vi "Initialize.vi"(0 "ToneCloud in":refnum<class "Tone Cloud.lvclass">, 1 "Filter in":refnum<class "Filter.lvclass">, 5 "Level in":refnum<class "Level.lvclass">, 7 "Fs (Hz)":dbl, 9 "Npts":i32, 11 "error in (no error)":errorcluster, 13 "Channel Name":string) -> (3 "Filter out":refnum<class "Filter.lvclass">, 4 "ToneCloud out":refnum<class "Tone Cloud.lvclass">, 6 "Level out":refnum<class "Level.lvclass">, 15 "error out":errorcluster)   [LabVIEW 2020, in "Tone Cloud.lvclass"]
uses:
  Tone Cloud.lvclass
  Level/Level.lvclass
  Filter/Filter.lvclass
  Tone Cloud.lvclass/Tone Cloud.ctl
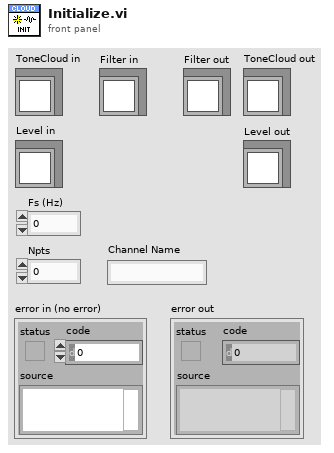
[diagram p1: front panel]
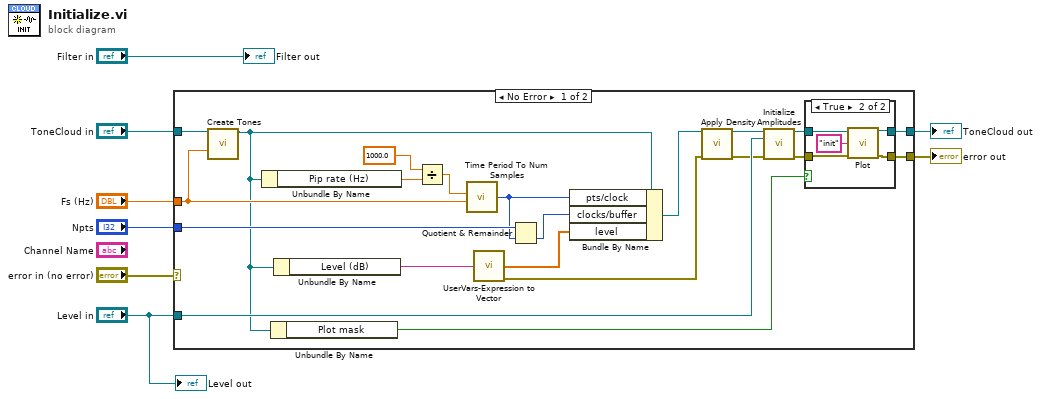
[diagram p0: block diagram]
diagram:
  n1 = case shown="No Error" "error in (no error)" {
    selector: "error in (no error)" -> [_ w37]
    tunnel: "ToneCloud in" -> [w29 w38]
    tunnel: "Level in" -> [w19 _]
    tunnel: "Fs (Hz)" -> [w28 _]
    tunnel: "Npts" -> [w24 _]
    tunnel: [w13 w38] -> w3
    tunnel: [w11 w37] -> w2
    frame No Error {
      n2 = call "Create Tones.vi"("ToneCloud in"=w29, "Fs (Hz)"=w28) -> ("ToneCloud out"=w14:refnum<class "Tone Cloud.lvclass">)  [unwired: 12 in, 1 out]
      n3 = Unbundle By Name(w14) -> ("Pip rate (Hz)"=w27:dbl)
      n4 = Unbundle By Name(w14) -> ("Plot mask"=w9:bool)
      n5 = Unbundle By Name(w14) -> ("Level (dB)"=w21:string)
      n6 = Divide(x=1000.0, y=w27) -> (x/y=w25:dbl)
      n7 = call "Time Period To Num Samples.vi"("Duration (ms)"=w25, "Sampling rate (Hz)"=w28) -> ("Samples"=w23:i32)  [unwired: 5 in]
      n8 = call "UserVars-Expression to Vector.vi"("Expr"=w21) -> ("Values"=w20:dbl[], "error out"=w17:errorcluster)  [unwired: 13 in]
      n9 = Quotient & Remainder(x=w24, y=w23) -> (floor(x/y)=w22:i32)  [unwired: 1 out]
      n10 = Bundle By Name(cluster=w14, "pts/clock"=w23, "clocks/buffer"=w22, "level"=w20) -> (w18:refnum<class "Tone Cloud.lvclass">)
      n11 = call "Apply Density.vi"("ToneCloud in"=w18, "error in (no error)"=w17) -> ("ToneCloud out"=w15:refnum<class "Tone Cloud.lvclass">, "error out"=w16:errorcluster)  [unwired: 12 in]
      n12 = call "Initialize Amplitudes.vi"("ToneCloud in"=w15, "Level in"=w19, "error in (no error)"=w16) -> ("ToneCloud out"=w12:refnum<class "Tone Cloud.lvclass">, "error out"=w10:errorcluster)  [unwired: 11 in]
      n13 = case shown="True" w9 {
        tunnel: [w31 w35] -> w13
        tunnel: w12 -> [w31 w36]
        tunnel: [w30 w34] -> w11
        tunnel: w10 -> [w30 w33]
        frame False {
        }
        frame True {
          n14 = call "Plot.vi"("ToneCloud in"=w36, "action"="init", "error in (no error)"=w33) -> ("ToneCloud out"=w35:refnum<class "Tone Cloud.lvclass">, "error out"=w34:errorcluster)  [unwired: 11 in]
        }
      }
    }
    frame Error {
    }
  }
  "error out" <- w2
  "ToneCloud out" <- w3
  "Level out" <- "Level in"
  "Filter out" <- "Filter in"
